vi "SVI_SerialSendAndReceiveChecksumWithACKNAK.vi"(4 "NAK":string="N", 5 "ACK":string="A", 6 "Retries":i32=50, 7 "Wait Time (ms)":u32=10, 8 "error in (no error)":errorcluster, 9 "Send Checksum":bool, 10 "Command":string, 11 "VISA Refnum in":refnum<visa-resource-name>) -> (0 "error out":errorcluster, 2 "Received":string, 3 "VISA resource name out":refnum<visa-resource-name>)   [LabVIEW 2014]
panel:
  out "Array 3":string[](array[string])
  out "ACK 2":string
  out "Array 2":string[](array[string])
  out "concatenated string":string
  out "Numeric Control 2":i32
  out "Array":u32[](array[numeric])
  out "Numeric Control":i32
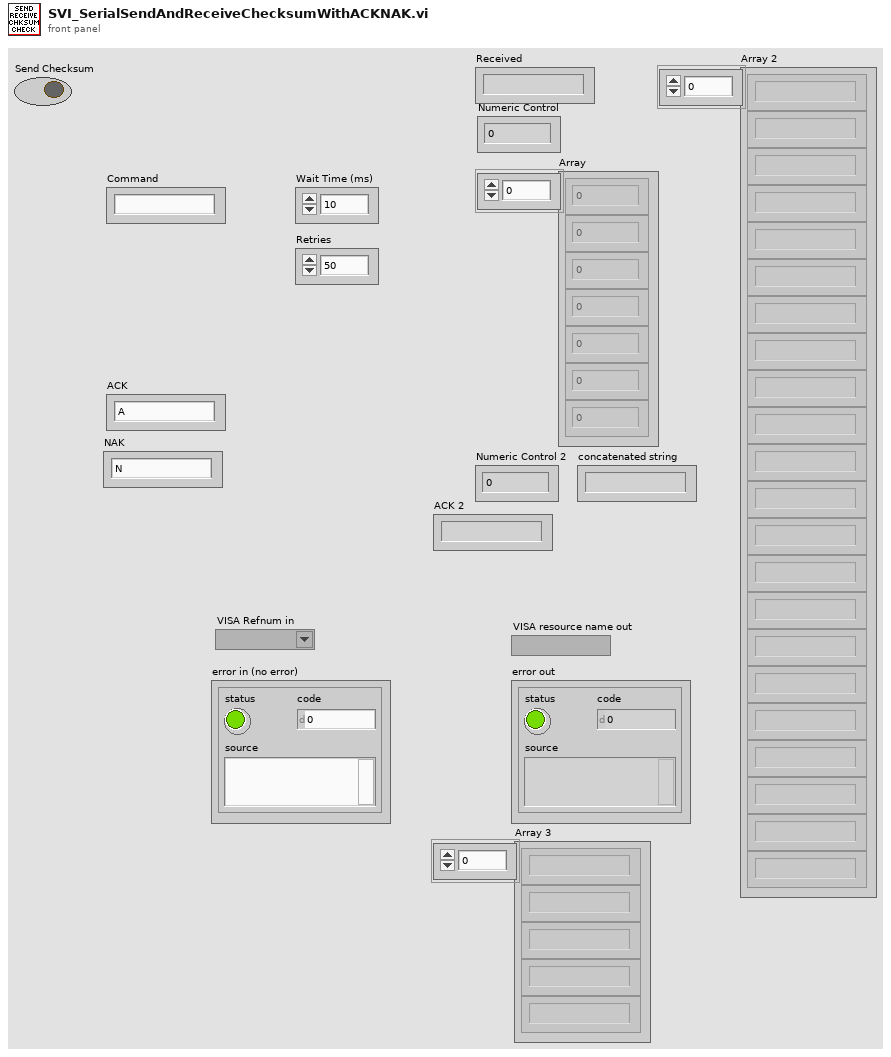
[diagram p1: front panel]
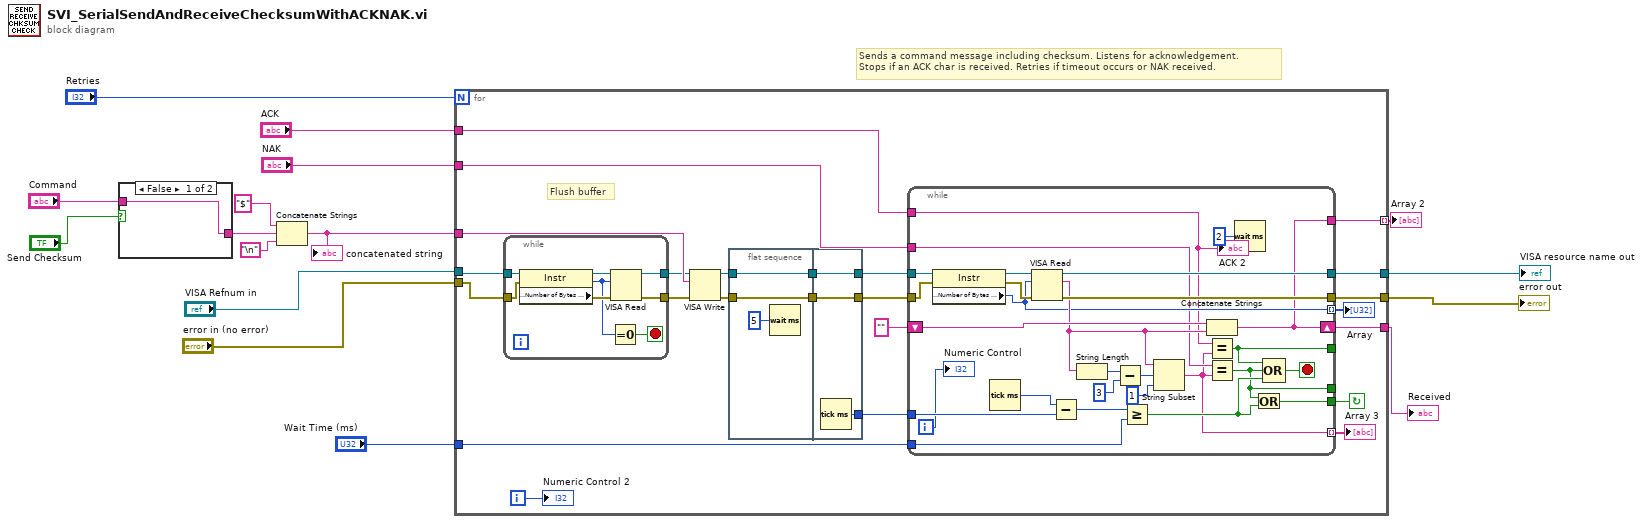
[diagram p0: block diagram]
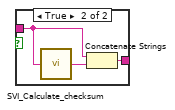
[diagram p2: hidden frame]
diagram:
  # "Sends a command message including checksum. Listens for acknowledgement.\nStops if an ACK char is received. Retries if timeout occurs or NAK received."
  n1 = case shown="False" "Send Checksum" {
    tunnel: [w17 w20] -> w12
    tunnel: "Command" -> [w17 w18]
    frame False {
    }
    frame True {
      n2 = call "SVI_Calculate_checksum.vi"("Message"=w18) -> ("Calculated checksum"=w19:string)
      n3 = Concatenate Strings(w18, w19) -> (w20:string)
    }
  }
  n4 = Concatenate Strings("$" ("string"), w12, "\n") -> (w13:string)
  "concatenated string" <- w13
  n5 = for {
    N: "Retries" -> [_]
    tunnel: w13 -> [w43]
    tunnel: "error in (no error)" -> [w23]
    tunnel: "VISA Refnum in" -> [w22]
    tunnel: "Wait Time (ms)" -> [w38]
    tunnel: "NAK" -> [w36]
    tunnel: "ACK" -> [w32]
    tunnel: [w35] -> w3
    tunnel: [w34] -> w7
    tunnel: [w33] -> w6
    tunnel: [w29] -> w4 mode=indexing
    i -> [w30]
    stop <- w37 continue-if-true
    # "Flush buffer"
    n6 = while {
      tunnel: w22 -> [w48]
      tunnel: [w47] -> w24
      tunnel: w23 -> [w49]
      tunnel: [w50] -> w25
      stop <- w46 stop-if-true
      n7 = property class="Instr"(reference=w48, error in=w49) -> (reference out=w52:refnum<visa-resource-name>, error out=w51:errorcluster, "Serial Settings:Number of Bytes at Serial Port"=w45:u32)
      n8 = Equal To 0?(x=w45) -> (x = 0?=w46:bool)
      n9 = VISA Read(VISA resource name=w52, byte count=w45, error in (no error)=w51) -> (VISA resource name out=w47:refnum<visa-resource-name>, error out=w50:errorcluster)  [unwired: 2 out]
    }
    n10 = VISA Write(VISA resource name=w24, write buffer=w43, error in (no error)=w25) -> (VISA resource name out=w42:refnum<visa-resource-name>, error out=w44:errorcluster)  [unwired: 1 out]
    n11 = flat-sequence {
      tunnel: w44 -> [w83]
      tunnel: w42 -> [w82]
      tunnel: [w83] -> w28
      tunnel: [w82] -> w27
      tunnel: [w85] -> w39
      tunnel: [w86] -> w40
      tunnel: w28 -> [w86]
      tunnel: w27 -> [w85]
      tunnel: [w84] -> w26
      frame #0 {
        n12 = Wait (ms)(milliseconds to wait=u32 5) -> ()  [unwired: 1 out]
      }
      frame #1 {
        n13 = Tick Count (ms)() -> (millisecond timer value=w84:u32)
      }
    }
    n14 = while {
      tunnel: w39 -> [w78]
      tunnel: [w76] -> w34
      shift-right: [w63] -> w33
      shift-left: "" -> [w74]
      tunnel: w26 -> [w72]
      tunnel: w40 -> [w77]
      tunnel: [w75] -> w35
      tunnel: w38 -> [w70]
      tunnel: [w62] -> w37
      tunnel: [w69] -> w31 mode=indexing
      tunnel: w36 -> [w68]
      tunnel: w32 -> [w67]
      tunnel: [w63] -> w29
      tunnel: [w60] -> _
      tunnel: [w59] -> _
      tunnel: [w57] -> w21 mode=indexing
      i -> [w64]
      stop <- w66 stop-if-true
      n15 = property class="Instr"(reference=w78, error in=w77) -> (reference out=w80:refnum<visa-resource-name>, error out=w79:errorcluster, "Serial Settings:Number of Bytes at Serial Port"=w69:u32)
      n16 = Tick Count (ms)() -> (millisecond timer value=w73:u32)
      n17 = VISA Read(VISA resource name=w80, byte count=w69, error in (no error)=w79) -> (VISA resource name out=w76:refnum<visa-resource-name>, read buffer=w71:string, error out=w75:errorcluster)  [unwired: 1 out]
      n18 = Subtract(x=w73, y=w72) -> (x-y=w61:u32)
      n19 = String Length(string=w71) -> (length=w56:i32)
      n20 = Subtract(x=w56, y=3) -> (x-y=w55:i32)
      n21 = Greater Or Equal?(x=w61, y=w70) -> (x >= y?=w65:bool)
      n22 = String Subset(string=w71, offset (0)=w55, length (rest)=1 ("length (rest)")) -> (substring=w57:string)
      n23 = Concatenate Strings(w74, w71) -> (w63:string)
      n24 = Equal?(x=w67, y=w57) -> (x = y?=w60:bool)
      n25 = Equal?(x=w68, y=w57) -> (x = y?=w59:bool)
      n26 = Wait (ms)(milliseconds to wait=u32 2) -> ()  [unwired: 1 out]
      n27 = Or(x=w59, y=w65) -> (x .or. y?=w62:bool)
      n28 = Compound Arithmetic op=OR(w60, w59, w65) -> (w66:bool)
      "Numeric Control" <- w64
      "ACK 2" <- w67
    }
    "Array" <- w31
    "Array 3" <- w21
    "Numeric Control 2" <- w30
  }
  "error out" <- w3
  "VISA resource name out" <- w7
  "Received" <- w6
  "Array 2" <- w4
